vi "CAN自动测试.vi"(10 "选择?":bool) -> ()   [LabVIEW 2010]
uses:
  全局量/试验配置信息.vi
  全局量/自动测试结果.vi
panel:
  in  "同步_2":i32
  in  "同步_1":i32
  out "结束?":bool
  in  "CAN_4_4":u16
  in  "CAN_4_3":u16
  in  "CAN_4_2":u16
  in  "CAN_4_1":u16
  in  "CAN_3_4":u16
  in  "CAN_3_3":u16
  in  "CAN_3_2":u16
  in  "CAN_3_1":u16
  in  "CAN_2_4":u16
  in  "CAN_2_3":u16
  in  "CAN_2_2":u16
  in  "CAN_2_1":u16
  in  "CAN_1_4":u16
  in  "CAN_1_3":u16
  in  "CAN_1_2":u16
  in  "CAN_1_1":u16
  # "CAN1"
  # "CAN2"
  # "CAN3"
  # "CAN4"
  # "测试结论："
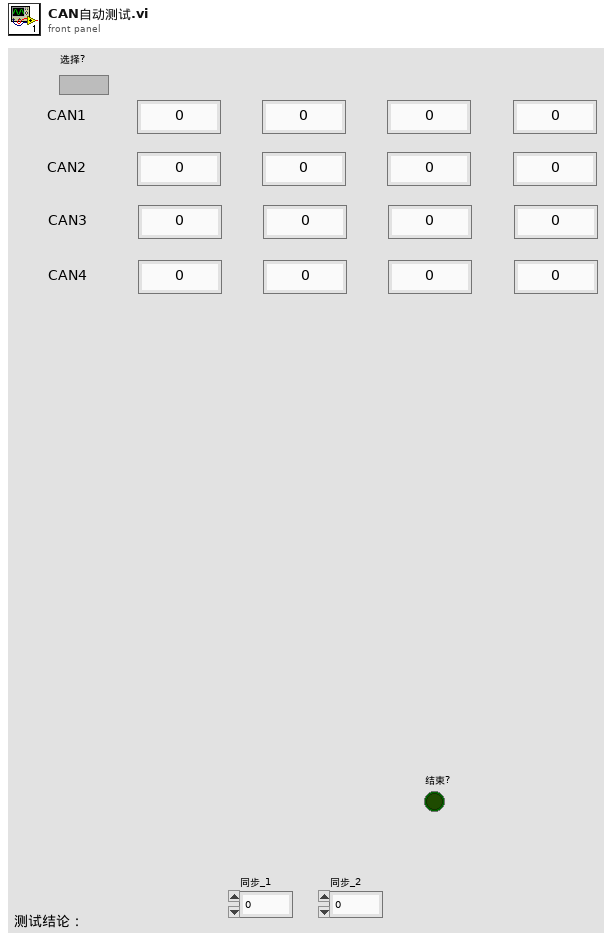
[diagram p1: front panel]
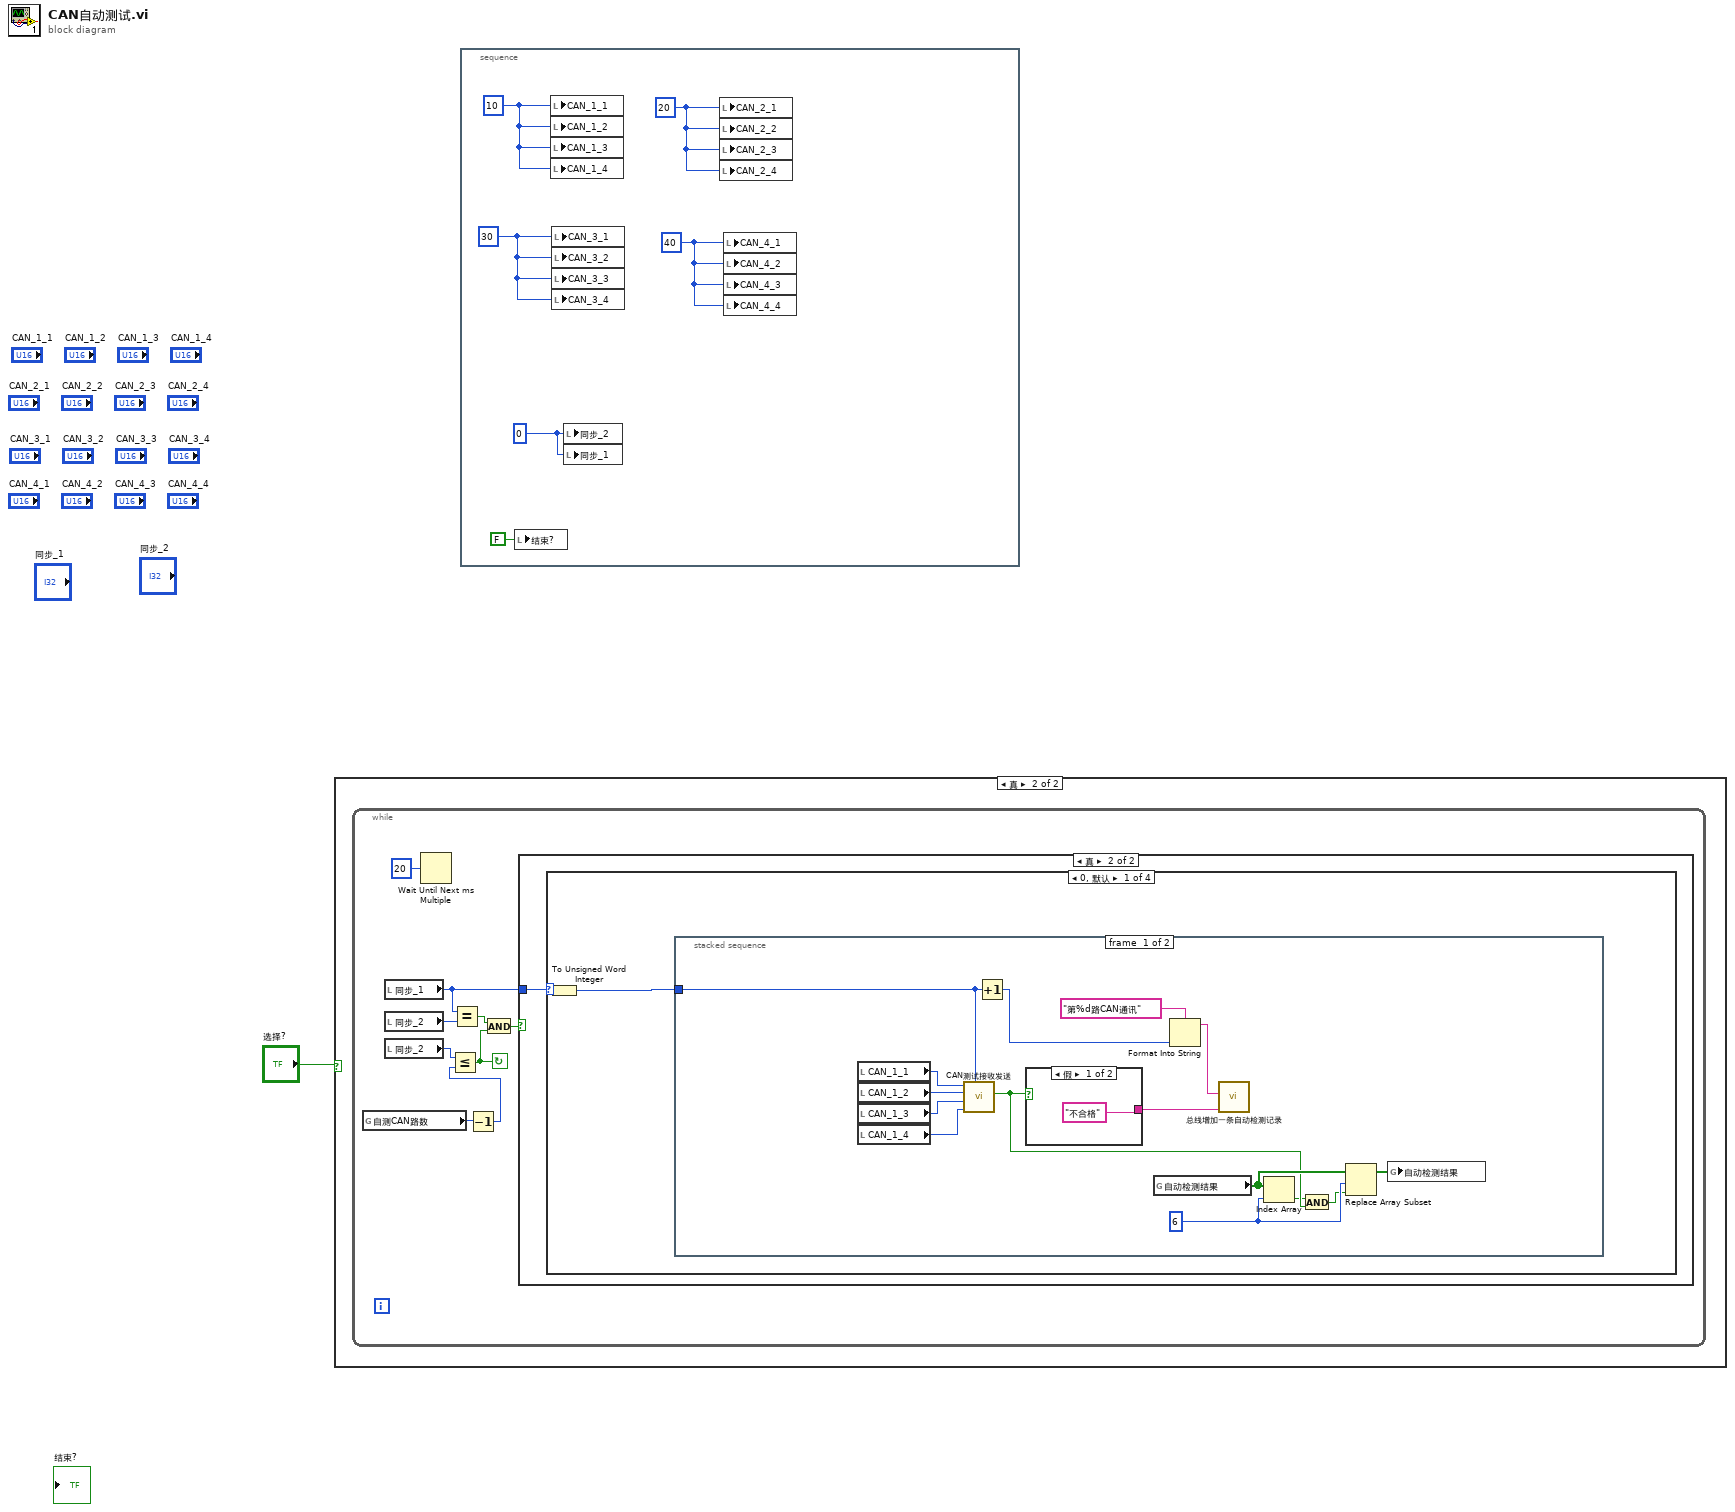
[diagram p0: block diagram]
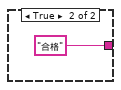
[diagram p4: hidden frame]
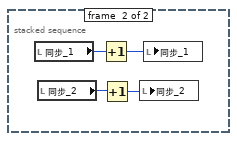
[diagram p5: hidden frame]
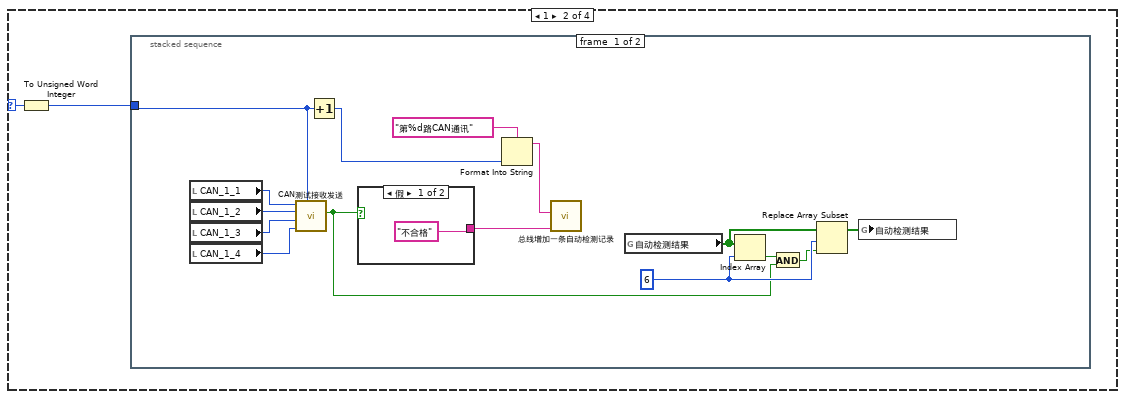
[diagram p6: hidden frame]
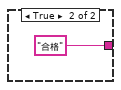
[diagram p7: hidden frame]
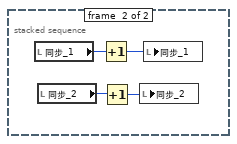
[diagram p8: hidden frame]
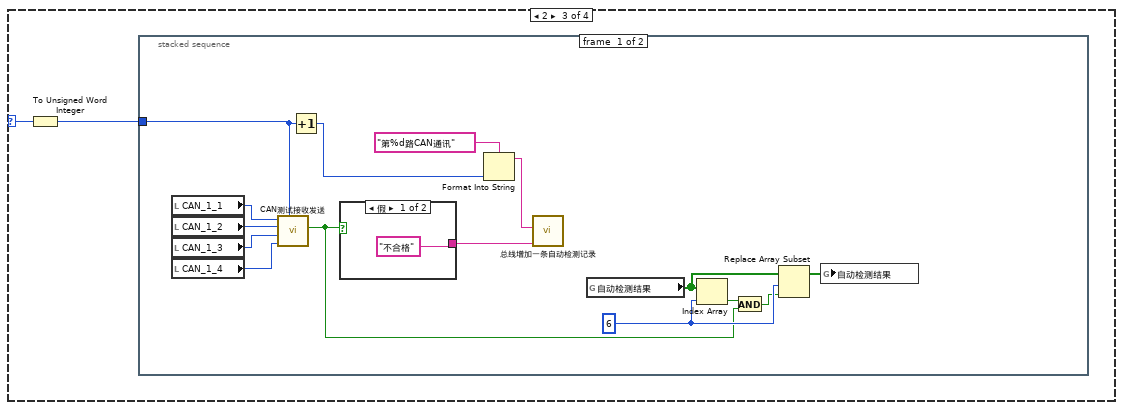
[diagram p9: hidden frame]
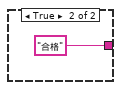
[diagram p10: hidden frame]
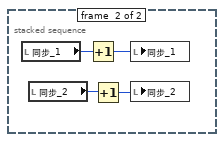
[diagram p11: hidden frame]
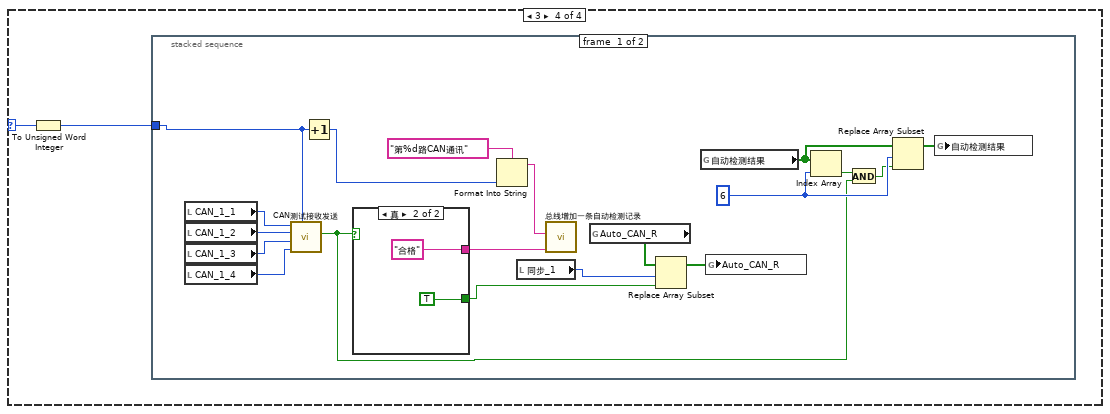
[diagram p12: hidden frame]
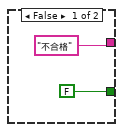
[diagram p13: hidden frame]
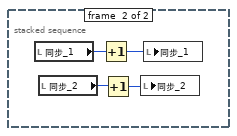
[diagram p14: hidden frame]
diagram:
  n1 = case shown="真" "选择?" {
    frame False {
    }
    frame True {
      n2 = while {
        stop <- w4 continue-if-true
        n3 = global read "试验配置信息.vi" "自测CAN路数"() -> (w3:i32)
        n4 = local read "同步_1"() -> (w10:i32)
        n5 = local read "同步_2"() -> (w7:i32)
        n6 = local read "同步_2"() -> (w9:i32)
        n7 = Wait Until Next ms Multiple(millisecond multiple=u32 20 ("毫秒倍数")) -> ()  [unwired: 1 out]
        n8 = Equal?(x=w10, y=w7) -> (x = y?=w5:bool)
        n9 = Decrement(x=w3) -> (x-1=w2:i32)
        n10 = Less Or Equal?(x=w9, y=w2) -> (x <= y?=w4:bool)
        n11 = And(x=w5, y=w4) -> (x .and. y?=w6:bool)
        n12 = case shown="真" w6 {
          tunnel: w10 -> [_ w11]
          frame False {
          }
          frame True {
            n13 = case shown="0, 默认" w11 {
              selector: w11 -> [w12 w36 w59 w82]
              frame 0, Default {
                n14 = To Unsigned Word Integer(number=w12) -> (unsigned 16bit integer=w13:u16)
                n15 = stacked-sequence {
                  tunnel: w13 -> [w24 _]
                  frame #0 {
                    w17 = 6 ("索引")
                    n16 = local read "CAN_1_1"() -> (w25:u16)
                    n17 = local read "CAN_1_2"() -> (w26:u16)
                    n18 = local read "CAN_1_3"() -> (w27:u16)
                    n19 = local read "CAN_1_4"() -> (w28:u16)
                    n20 = call "CAN测试接收发送.vi"("Order"=w24, "data_4"=w28, "data_3"=w27, "data_2"=w26, "data_1"=w25) -> ("成功？"=w16:bool)  [unwired: 5 in, 1 out]
                    n21 = Increment(x=w24) -> (x+1=w22:u16)
                    n22 = case shown="假" w16 {
                      tunnel: ["不合格" "合格"] -> w20
                      frame False {
                      }
                      frame True {
                      }
                    }
                    n23 = global read "试验配置信息.vi" "自动检测结果"() -> (w18:bool[])
                    n24 = Format Into String(format string="第%d路CAN通讯", w22) -> (resulting string=w21:string)  [unwired: 2 in, 1 out]
                    n25 = call "总线增加一条自动检测记录.vi"("测试结果"=w20, "测试内容"=w21) -> ()  [unwired: 10 in]
                    n26 = Index Array(array=w18, index=w17) -> (element=w15:bool)
                    n27 = And(x=w15, y=w16) -> (x .and. y?=w14:bool)
                    n28 = Replace Array Subset(array=w18, new element=w14, index=w17) -> (w19:bool[])
                    n29 = global write "试验配置信息.vi" "自动检测结果"(w19) -> ()
                  }
                  frame #1 {
                    n30 = local read "同步_1"() -> (w33:i32)
                    n31 = local read "同步_2"() -> (w31:i32)
                    n32 = Increment(x=w33) -> (x+1=w34:i32)
                    n33 = Increment(x=w31) -> (x+1=w32:i32)
                    n34 = local write "同步_2"(w32) -> ()
                    n35 = local write "同步_1"(w34) -> ()
                  }
                }
              }
              frame 1 {
                n36 = To Unsigned Word Integer(number=w36) -> (unsigned 16bit integer=w35:u16)
                n37 = stacked-sequence {
                  tunnel: w35 -> [w43 _]
                  frame #0 {
                    w40 = 6 ("索引")
                    n38 = local read "CAN_1_1"() -> (w48:u16)
                    n39 = local read "CAN_1_2"() -> (w49:u16)
                    n40 = local read "CAN_1_3"() -> (w50:u16)
                    n41 = local read "CAN_1_4"() -> (w51:u16)
                    n42 = call "CAN测试接收发送.vi"("Order"=w43, "data_4"=w51, "data_3"=w50, "data_2"=w49, "data_1"=w48) -> ("成功？"=w37:bool)  [unwired: 5 in, 1 out]
                    n43 = Increment(x=w43) -> (x+1=w46:u16)
                    n44 = case shown="假" w37 {
                      tunnel: ["不合格" "合格"] -> w44
                      frame False {
                      }
                      frame True {
                      }
                    }
                    n45 = Format Into String(format string="第%d路CAN通讯", w46) -> (resulting string=w45:string)  [unwired: 2 in, 1 out]
                    n46 = call "总线增加一条自动检测记录.vi"("测试结果"=w44, "测试内容"=w45) -> ()  [unwired: 10 in]
                    n47 = global read "试验配置信息.vi" "自动检测结果"() -> (w41:bool[])
                    n48 = Index Array(array=w41, index=w40) -> (element=w39:bool)
                    n49 = And(x=w39, y=w37) -> (x .and. y?=w38:bool)
                    n50 = Replace Array Subset(array=w41, new element=w38, index=w40) -> (w42:bool[])
                    n51 = global write "试验配置信息.vi" "自动检测结果"(w42) -> ()
                  }
                  frame #1 {
                    n52 = local read "同步_1"() -> (w56:i32)
                    n53 = local read "同步_2"() -> (w55:i32)
                    n54 = Increment(x=w56) -> (x+1=w57:i32)
                    n55 = Increment(x=w55) -> (x+1=w54:i32)
                    n56 = local write "同步_2"(w54) -> ()
                    n57 = local write "同步_1"(w57) -> ()
                  }
                }
              }
              frame 2 {
                n58 = To Unsigned Word Integer(number=w59) -> (unsigned 16bit integer=w58:u16)
                n59 = stacked-sequence {
                  tunnel: w58 -> [w66 _]
                  frame #0 {
                    w63 = 6 ("索引")
                    n60 = local read "CAN_1_1"() -> (w71:u16)
                    n61 = local read "CAN_1_2"() -> (w72:u16)
                    n62 = local read "CAN_1_3"() -> (w73:u16)
                    n63 = local read "CAN_1_4"() -> (w74:u16)
                    n64 = call "CAN测试接收发送.vi"("Order"=w66, "data_4"=w74, "data_3"=w73, "data_2"=w72, "data_1"=w71) -> ("成功？"=w60:bool)  [unwired: 5 in, 1 out]
                    n65 = Increment(x=w66) -> (x+1=w69:u16)
                    n66 = case shown="假" w60 {
                      tunnel: ["不合格" "合格"] -> w67
                      frame False {
                      }
                      frame True {
                      }
                    }
                    n67 = Format Into String(format string="第%d路CAN通讯", w69) -> (resulting string=w68:string)  [unwired: 2 in, 1 out]
                    n68 = call "总线增加一条自动检测记录.vi"("测试结果"=w67, "测试内容"=w68) -> ()  [unwired: 10 in]
                    n69 = global read "试验配置信息.vi" "自动检测结果"() -> (w64:bool[])
                    n70 = Index Array(array=w64, index=w63) -> (element=w62:bool)
                    n71 = And(x=w62, y=w60) -> (x .and. y?=w61:bool)
                    n72 = Replace Array Subset(array=w64, new element=w61, index=w63) -> (w65:bool[])
                    n73 = global write "试验配置信息.vi" "自动检测结果"(w65) -> ()
                  }
                  frame #1 {
                    n74 = local read "同步_1"() -> (w79:i32)
                    n75 = local read "同步_2"() -> (w77:i32)
                    n76 = Increment(x=w79) -> (x+1=w80:i32)
                    n77 = Increment(x=w77) -> (x+1=w78:i32)
                    n78 = local write "同步_1"(w80) -> ()
                    n79 = local write "同步_2"(w78) -> ()
                  }
                }
              }
              frame 3 {
                n80 = To Unsigned Word Integer(number=w82) -> (unsigned 16bit integer=w81:u16)
                n81 = stacked-sequence {
                  tunnel: w81 -> [w93 _]
                  frame #0 {
                    w86 = 6 ("索引")
                    n82 = local read "CAN_1_1"() -> (w98:u16)
                    n83 = local read "CAN_1_2"() -> (w99:u16)
                    n84 = local read "CAN_1_3"() -> (w100:u16)
                    n85 = local read "CAN_1_4"() -> (w101:u16)
                    n86 = call "CAN测试接收发送.vi"("Order"=w93, "data_4"=w101, "data_3"=w100, "data_2"=w99, "data_1"=w98) -> ("成功？"=w83:bool)  [unwired: 5 in, 1 out]
                    n87 = Increment(x=w93) -> (x+1=w96:u16)
                    n88 = case shown="真" w83 {
                      tunnel: ["不合格" "合格"] -> w94
                      tunnel: [FALSE TRUE] -> w89
                      frame False {
                      }
                      frame True {
                      }
                    }
                    n89 = Format Into String(format string="第%d路CAN通讯", w96) -> (resulting string=w95:string)  [unwired: 2 in, 1 out]
                    n90 = local read "同步_1"() -> (w90:i32)
                    n91 = call "总线增加一条自动检测记录.vi"("测试结果"=w94, "测试内容"=w95) -> ()  [unwired: 10 in]
                    n92 = global read "自动测试结果.vi" "Auto_CAN_R"() -> (w92:bool[])
                    n93 = Replace Array Subset(array=w92, new element=w89, index=w90) -> (w91:bool[])
                    n94 = global read "试验配置信息.vi" "自动检测结果"() -> (w87:bool[])
                    n95 = global write "自动测试结果.vi" "Auto_CAN_R"(w91) -> ()
                    n96 = Index Array(array=w87, index=w86) -> (element=w85:bool)
                    n97 = And(x=w85, y=w83) -> (x .and. y?=w84:bool)
                    n98 = Replace Array Subset(array=w87, new element=w84, index=w86) -> (w88:bool[])
                    n99 = global write "试验配置信息.vi" "自动检测结果"(w88) -> ()
                  }
                  frame #1 {
                    n100 = local read "同步_1"() -> (w109:i32)
                    n101 = local read "同步_2"() -> (w106:i32)
                    n102 = Increment(x=w109) -> (x+1=w108:i32)
                    n103 = Increment(x=w106) -> (x+1=w107:i32)
                    n104 = local write "同步_2"(w107) -> ()
                    n105 = local write "同步_1"(w108) -> ()
                  }
                }
              }
            }
          }
        }
      }
    }
  }
  n106 = stacked-sequence {
    frame #0 {
      w110 = u16 30 ("CAN_R_3_1")
      w111 = u16 40 ("CAN_R_4_1")
      w112 = u16 20 ("CAN_R_2_1")
      w113 = u16 10 ("CAN_R_1_1")
      w114 = 0 ("同步_2")
      n107 = local write "结束?"(FALSE ("结束?")) -> ()
      n108 = local write "CAN_1_1"(w113) -> ()
      n109 = local write "CAN_1_2"(w113) -> ()
      n110 = local write "CAN_1_3"(w113) -> ()
      n111 = local write "CAN_1_4"(w113) -> ()
      n112 = local write "CAN_3_1"(w110) -> ()
      n113 = local write "CAN_3_2"(w110) -> ()
      n114 = local write "CAN_3_3"(w110) -> ()
      n115 = local write "CAN_3_4"(w110) -> ()
      n116 = local write "同步_2"(w114) -> ()
      n117 = local write "同步_1"(w114) -> ()
      n118 = local write "CAN_2_1"(w112) -> ()
      n119 = local write "CAN_2_2"(w112) -> ()
      n120 = local write "CAN_2_3"(w112) -> ()
      n121 = local write "CAN_2_4"(w112) -> ()
      n122 = local write "CAN_4_1"(w111) -> ()
      n123 = local write "CAN_4_2"(w111) -> ()
      n124 = local write "CAN_4_3"(w111) -> ()
      n125 = local write "CAN_4_4"(w111) -> ()
    }
  }
